vi "formatReportImage.vi"(6 "Images Same?":bool, 8 "error in (no error)":errorcluster, 11 "Image Array":cluster{"Image Data":T1, "ImageType":string}[](array[cluster])) -> (0 "error out":errorcluster, 3 "Report String":string)   [LabVIEW 2018, in "Image_Diff.lvlib"]
uses:
  Image_Diff.lvlib
  <vilib>/picture/picture.llb/imagedata.ctl
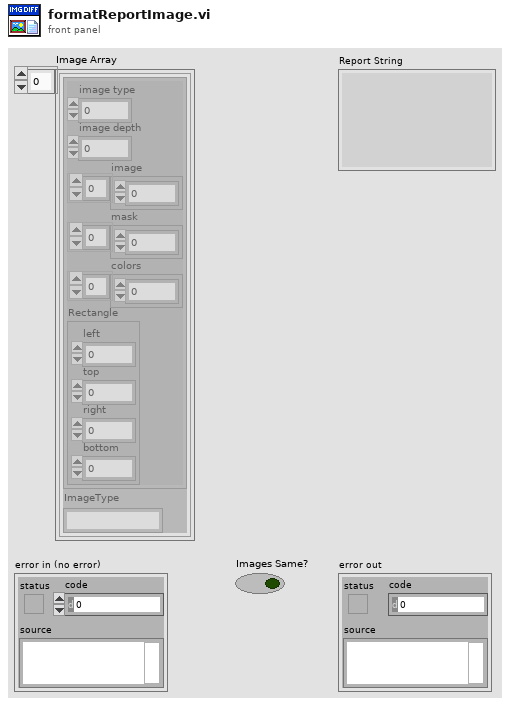
[diagram p1: front panel]
types:
  T1 = typedef "imagedata.ctl" = cluster{"image type":i32, "image depth":i32, "image":u8[], "mask":u8[], "colors":u32[], "Rectangle":cluster{"left":i16, "top":i16, "right":i16, "bottom":i16}}
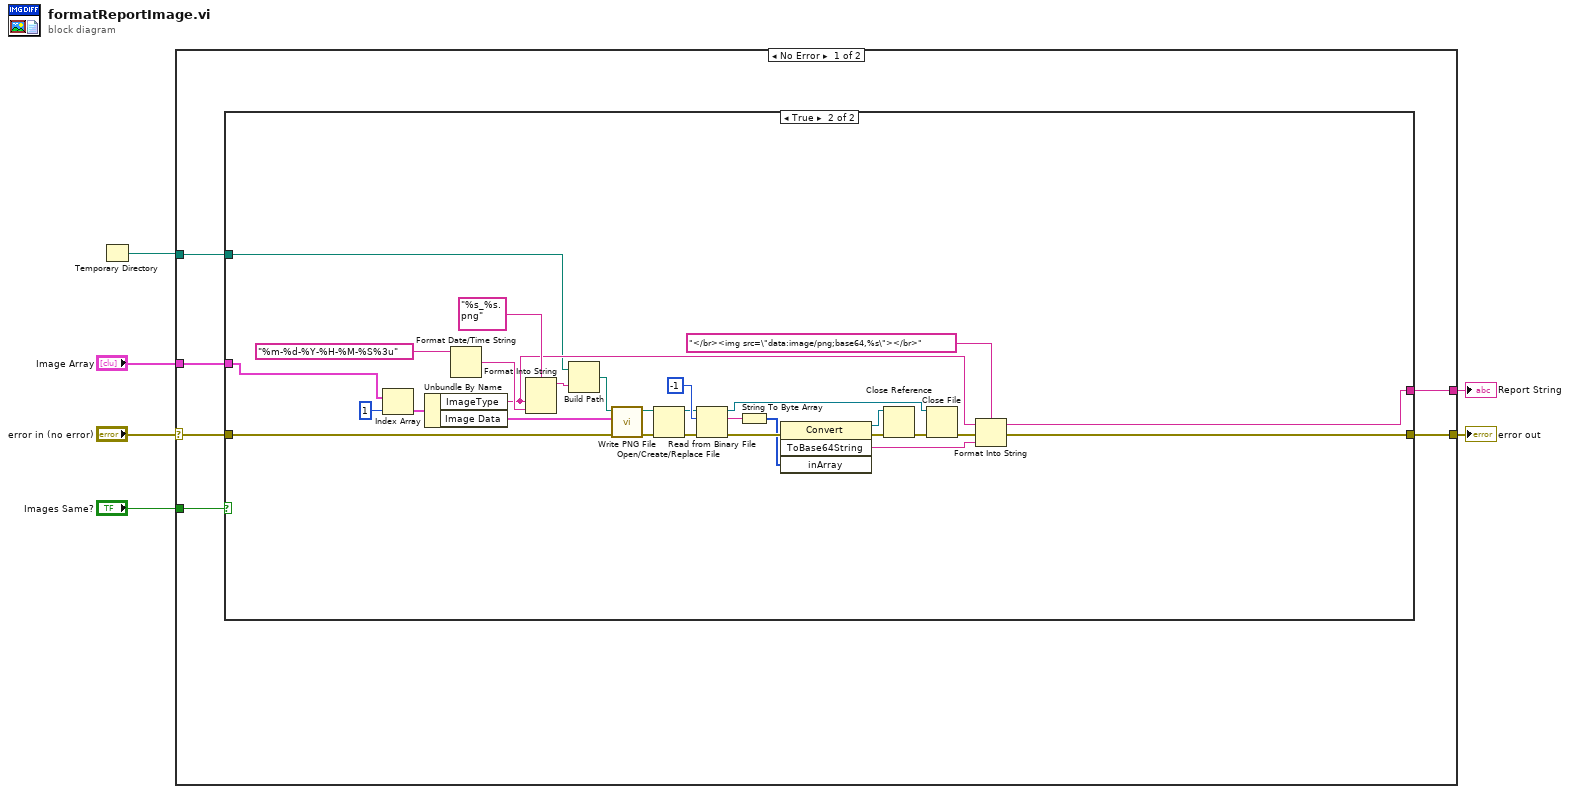
[diagram p0: block diagram]
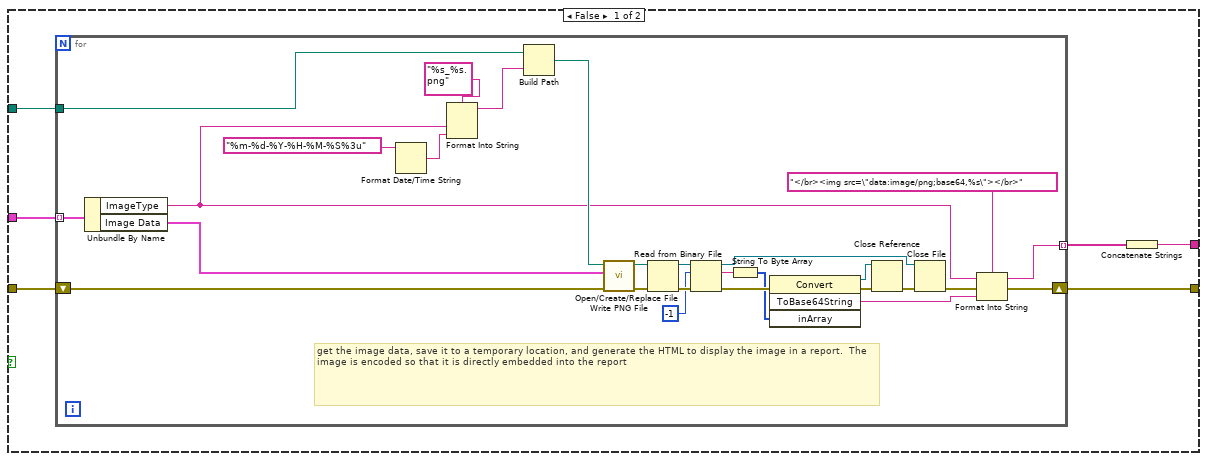
[diagram p2: hidden frame]
diagram:
  n1 = Temporary Directory() -> (w3:path)
  n2 = case shown="No Error" "error in (no error)" {
    selector: "error in (no error)" -> [w10 w75]
    tunnel: [w12 _] -> w6
    tunnel: [w11 w75] -> w5
    tunnel: w3 -> [w9 _]
    tunnel: "Image Array" -> [w8 _]
    tunnel: "Images Same?" -> [w7 _]
    frame No Error {
      n3 = case shown="True" w7 {
        tunnel: [w18 w46] -> w12
        tunnel: [w16 w47] -> w11
        tunnel: w10 -> [w15 w48]
        tunnel: w9 -> [w14 w52]
        tunnel: w8 -> [w13 w51]
        frame False {
          n4 = for {
            tunnel: [w44] -> w17 mode=indexing
            shift-right: [w26] -> w16
            shift-left: w15 -> [w23]
            tunnel: w14 -> [w25]
            tunnel: w13 -> [w24] mode=indexing
            # "get the image data, save it to a temporary location, and generate the HTML to display the image in a report.  The image is encoded so that it is directly embedded into the report"
            n5 = Unbundle By Name(w24) -> ("ImageType"=w19:string, "Image Data"=w21:T1)
            n6 = Format Date/Time String(time format string (%c)="%m-%d-%Y-%H-%M-%S%3u") -> (date/time string=w41:string)  [unwired: 2 in]
            n7 = Format Into String(format string="%s_%s.png", w19, w41) -> (resulting string=w42:string)  [unwired: 2 in, 1 out]
            n8 = Build Path(base path=w25, name or relative path=w42) -> (appended path=w22:path)
            n9 = call <vilib>:"Write PNG File.vi"("error in (no error)"=w23, "image data"=w21, "path to PNG file"=w22) -> ("error out"=w29:errorcluster, "path"=w28:path)  [unwired: 7 in]
            n10 = Open/Create/Replace File(file path (use dialog)=w28, error in=w29) -> (refnum out=w34:refnum<file>, error out=w39:errorcluster)  [unwired: 4 in, 1 out]
            n11 = Read from Binary File(8:w39, 10:-1 ("count (1)"), 11:w34) -> (0:w38:errorcluster, 2:w36:string, 3:w37:refnum<file>)  [unwired: 3 in, 1 out]
            n12 = String To Byte Array(string=w36) -> (unsigned byte array=w33:u8[])
            n13 = invoke class="Convert" method="ToBase64String"(error in=w38, "inArray"=w33) -> (reference out=w32:refnum<k24>, error out=w31:errorcluster, "ToBase64String"=w20:string)  [unwired: 2 in, 1 out]
            n14 = Close Reference(reference=w32, error in (no error)=w31) -> (error out=w30:errorcluster)
            n15 = Close File(refnum=w37, error in=w30) -> (error out=w27:errorcluster)  [unwired: 1 out]
            n16 = Format Into String(format string="</br><img src=\"data:image/png;base64,%s\"></br>", initial string=w19, error in=w27, w20) -> (resulting string=w44:string, error out=w26:errorcluster)
          }
          n17 = Concatenate Strings(w17) -> (w18:string)
        }
        frame True {
          n18 = Index Array(array=w51, index=1) -> (element=w49:cluster{"Image Data":T1, "ImageType":string})
          n19 = Unbundle By Name(w49) -> ("ImageType"=w53:string, "Image Data"=w55:T1)
          n20 = Format Date/Time String(time format string (%c)="%m-%d-%Y-%H-%M-%S%3u") -> (date/time string=w71:string)  [unwired: 2 in]
          n21 = Format Into String(format string="%s_%s.png", w53, w71) -> (resulting string=w72:string)  [unwired: 2 in, 1 out]
          n22 = Build Path(base path=w52, name or relative path=w72) -> (appended path=w56:path)
          n23 = call <vilib>:"Write PNG File.vi"("error in (no error)"=w48, "image data"=w55, "path to PNG file"=w56) -> ("error out"=w59:errorcluster, "path"=w58:path)  [unwired: 7 in]
          n24 = Open/Create/Replace File(file path (use dialog)=w58, error in=w59) -> (refnum out=w64:refnum<file>, error out=w69:errorcluster)  [unwired: 4 in, 1 out]
          n25 = Read from Binary File(8:w69, 10:-1 ("count (1)"), 11:w64) -> (0:w68:errorcluster, 2:w66:string, 3:w67:refnum<file>)  [unwired: 3 in, 1 out]
          n26 = String To Byte Array(string=w66) -> (unsigned byte array=w63:u8[])
          n27 = invoke class="Convert" method="ToBase64String"(error in=w68, "inArray"=w63) -> (reference out=w62:refnum<k24>, error out=w61:errorcluster, "ToBase64String"=w54:string)  [unwired: 2 in, 1 out]
          n28 = Close Reference(reference=w62, error in (no error)=w61) -> (error out=w60:errorcluster)
          n29 = Close File(refnum=w67, error in=w60) -> (error out=w57:errorcluster)  [unwired: 1 out]
          n30 = Format Into String(format string="</br><img src=\"data:image/png;base64,%s\"></br>", initial string=w53, error in=w57, w54) -> (resulting string=w46:string, error out=w47:errorcluster)
        }
      }
    }
    frame Error {
    }
  }
  "Report String" <- w6
  "error out" <- w5
